vi "play_speaker.vi"() -> ()   [LabVIEW 2014]
uses:
  <vilib>/Analysis/3filter.llb/Filter Passband Type.ctl
  <vilib>/FPGAPlugInAG/myRIO-1900/niLvFpga_Open_myRIO-1900.vi
  <vilib>/rvi/interface/common/dynamic/niFpgaDynamicAddResources.vi
  <vilib>/Analysis/3filter.llb/Butterworth Filter (DBL).vi
  <vilib>/Utility/error.llb/Error Cluster From Error Code.vi
  <vilib>/rvi/errors/niLvFpgaAdjustHostInterfaceError.vi
  <vilib>/FPGAPlugInAG/Dynamic/niLvFpga_Close_Dynamic.vi
  <vilib>/rvi/interface/nirviOpenFPGA/nirviOpenFPGA.xnode
  FPGA Bitfiles/project_FPGATarget_fpgalibrary_tD00r5qvfcc.lvbitx
  fpga_library.vi
  <vilib>/rvi/interface/nirviMethod/nirviMethod.xnode
  <vilib>/rvi/interface/nirviCloseFPGA/nirviCloseFPGA.xnode
  <vilib>/Analysis/NI_AALBase.lvlib
  <vilib>/rvi/errors/niLvFpgaMergeErrorWithErrorCode.vi
  <vilib>/FPGAPlugInAG/Dynamic/niLvFpga_ReadFifo_Dynamic.vi
  <vilib>/FPGAPlugInAG/Dynamic/niLvFpga_WriteFifo_Dynamic.vi
panel:
  out "Waveform Graph 3":u32[](graph)
  in  "volume":dbl=30.0 format="%#_13g"
  out "error out":errorcluster
  in  "Stop Button 2":bool
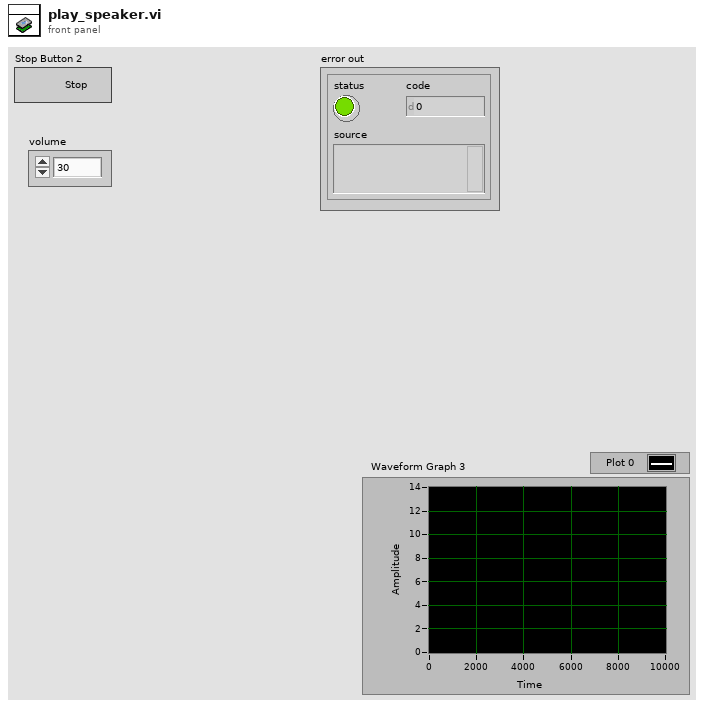
[diagram p1: front panel]
types:
  T1 = typedef "NI_AALBase.lvlib/Filter Passband Type.ctl" = enum32{"Lowpass", "Highpass", "Bandpass", "Bandstop"}
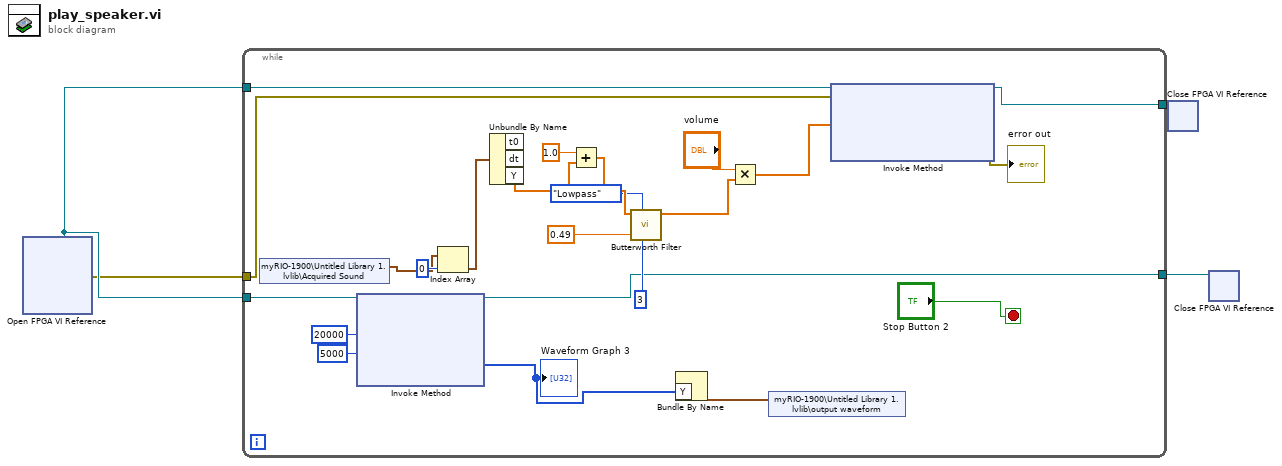
[diagram p0: block diagram]
diagram:
  n1 = xnode "Open FPGA VI Reference"() -> ("FPGA VI Reference Out"=w3:refnum<k20>, "error out"=w1:errorcluster)  [unwired: 2 in]
  n2 = while {
    tunnel: w3 -> [w26]
    tunnel: [w25] -> w4
    tunnel: w1 -> [w19]
    tunnel: w3 -> [w10]
    tunnel: [w9] -> w2
    stop <- "Stop Button 2" stop-if-true
    n3 = shared-variable "myRIO-1900\\Untitled Library 1.lvlib\\Acquired Sound"() -> (w11:waveform(dbl)[])  [unwired: 1 in, 1 out]
    n4 = xnode "Invoke Method"("FPGA VI Reference In"=w10, "Number of Elements"=u32 20000, "Timeout (ms)"=5000) -> ("FPGA VI Reference Out"=w9:refnum<k20>, "Data"=w6:u32[])  [unwired: 1 in, 2 out]
    "Waveform Graph 3" <- w6
    n5 = Index Array(array=w11, index=0) -> (element=w23:waveform(dbl))
    n6 = Unbundle By Name(w23) -> ("Y"=w21:dbl[])  [unwired: 2 out]
    n7 = Add(x=1.0, y=w21) -> (x+y=w18:dbl[])
    n8 = call-poly <vilib>:"Butterworth Filter.vi"("order"=3, "filter type"=Filter_Passband_Type."Lowpass", "low cutoff freq: fl"=0.49, "X"=w18) -> ("Filtered X"=w14:dbl[])  [unwired: 4 in, 1 out]
    n9 = Bundle By Name("Y"=w6) -> (w5:waveform(u32))  [unwired: 1 in]
    n10 = Multiply(x="volume", y=w14) -> (x*y=w12:dbl[])
    n11 = shared-variable "myRIO-1900\\Untitled Library 1.lvlib\\output waveform"(w5) -> ()  [unwired: 1 in, 1 out]
    n12 = xnode "Invoke Method"("FPGA VI Reference In"=w26, "error in"=w19, "Data"=w12) -> ("FPGA VI Reference Out"=w25:refnum<k20>, "error out"=→"error out":errorcluster)  [unwired: 1 in, 1 out]
  }
  n13 = xnode "Close FPGA VI Reference"("FPGA VI Reference In"=w4) -> ()  [unwired: 1 in, 1 out]
  n14 = xnode "Close FPGA VI Reference"("FPGA VI Reference In"=w2) -> ()  [unwired: 1 in, 1 out]
